vi "Main.vi"() -> ()   [LabVIEW 2015]
doc: "This example performs writes and reads on a serial port, as directed by the user. You can press the Write and Read buttons, and change the Read Count, while the example is running.\n\nThe parameters set for the serial port must match the parameters of the connected instrument or device. In this example, the Read Count parameter specifies the number of bytes that the serial port reads. If there were more bytes at the port than the specified number, those bytes would not be read. If there were less bytes at the port than the specified number, you would receive a timeout error.\n\nThis example expands upon the flow control options for XON and XOFF, allowing the user to choose those control characters. Also, the user can enable or disable a termination character. Some devices require a termination character in order to identify the end of command strings. Some devices send a termination character to signify the end of data to be read. This example shows how you can end the Read operation once a termination character is detected in the buffer and/or append a termination character at the end of the Write data."
uses:
  MPU-6050_states_machine_state.ctl
  <vilib>/Instr/_visa.llb/VISA Configure Serial Port (Instr).vi
panel:
  out "appended array":dbl[][](array[numeric])
  out "spreadsheet string":string
  out "x":dbl
  out "y":dbl
  out "z":dbl
  out "Pitch":dbl(knob) scale=0.0..360.0
  out "Roll":dbl(knob) scale=0.0..360.0
  out "Yaw":dbl(knob) scale=0.0..360.0
  out "read buffer":string
  in  "Save":bool
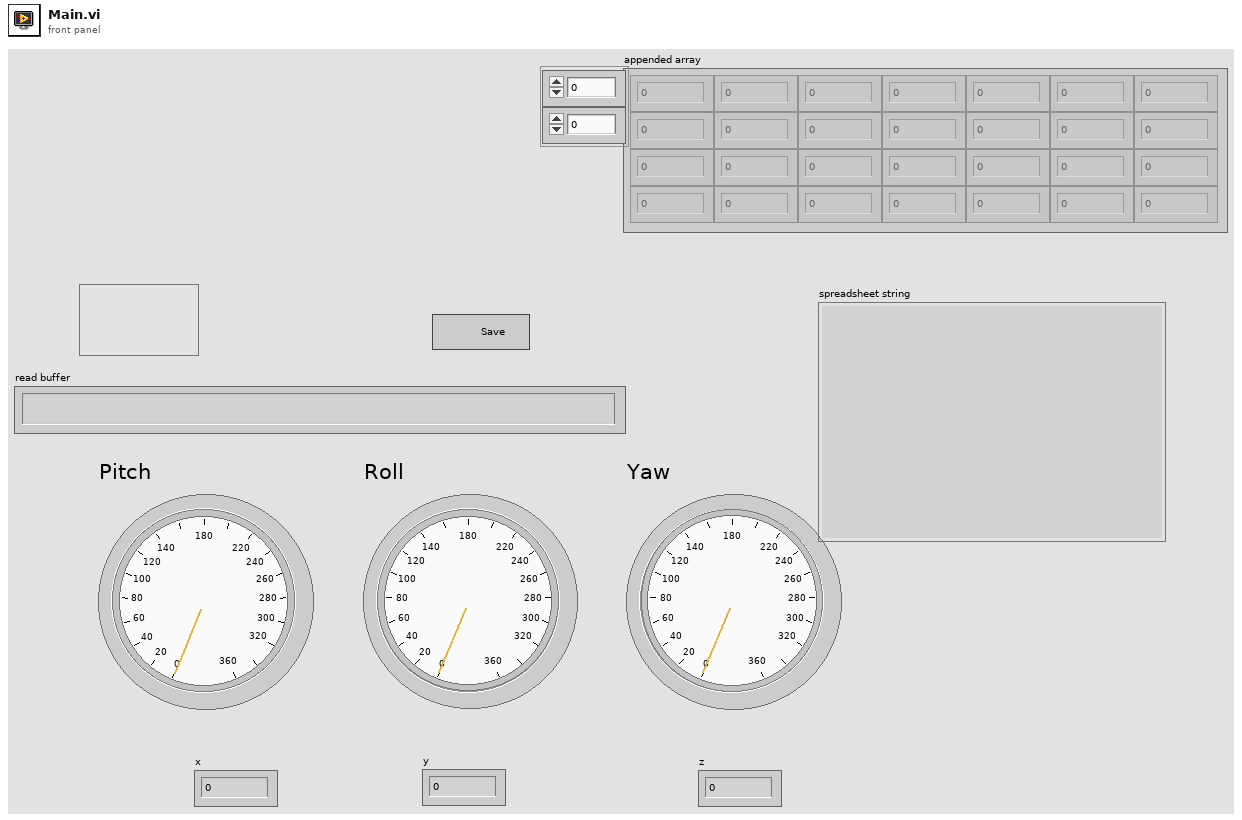
[diagram p1: front panel]
types:
  T1 = typedef "MPU-6050_states_machine_state.ctl" = enum16{"Initialize", "Calibrate", "Read", "Save", "Close", "Stop"}
  T2 = cluster{"VISA resource name":refnum<visa-resource-name>, "baud rate (9600)":u32, "Read buffer":string, "Byte count":u32, "GyroZ_bias":dbl, "GyraY_bias":dbl, "AccelX_bias":dbl, "AccelY_bias":dbl, "AccelZ_bias":dbl, "GyroX_bias":dbl, "Measurements":dbl[][]}
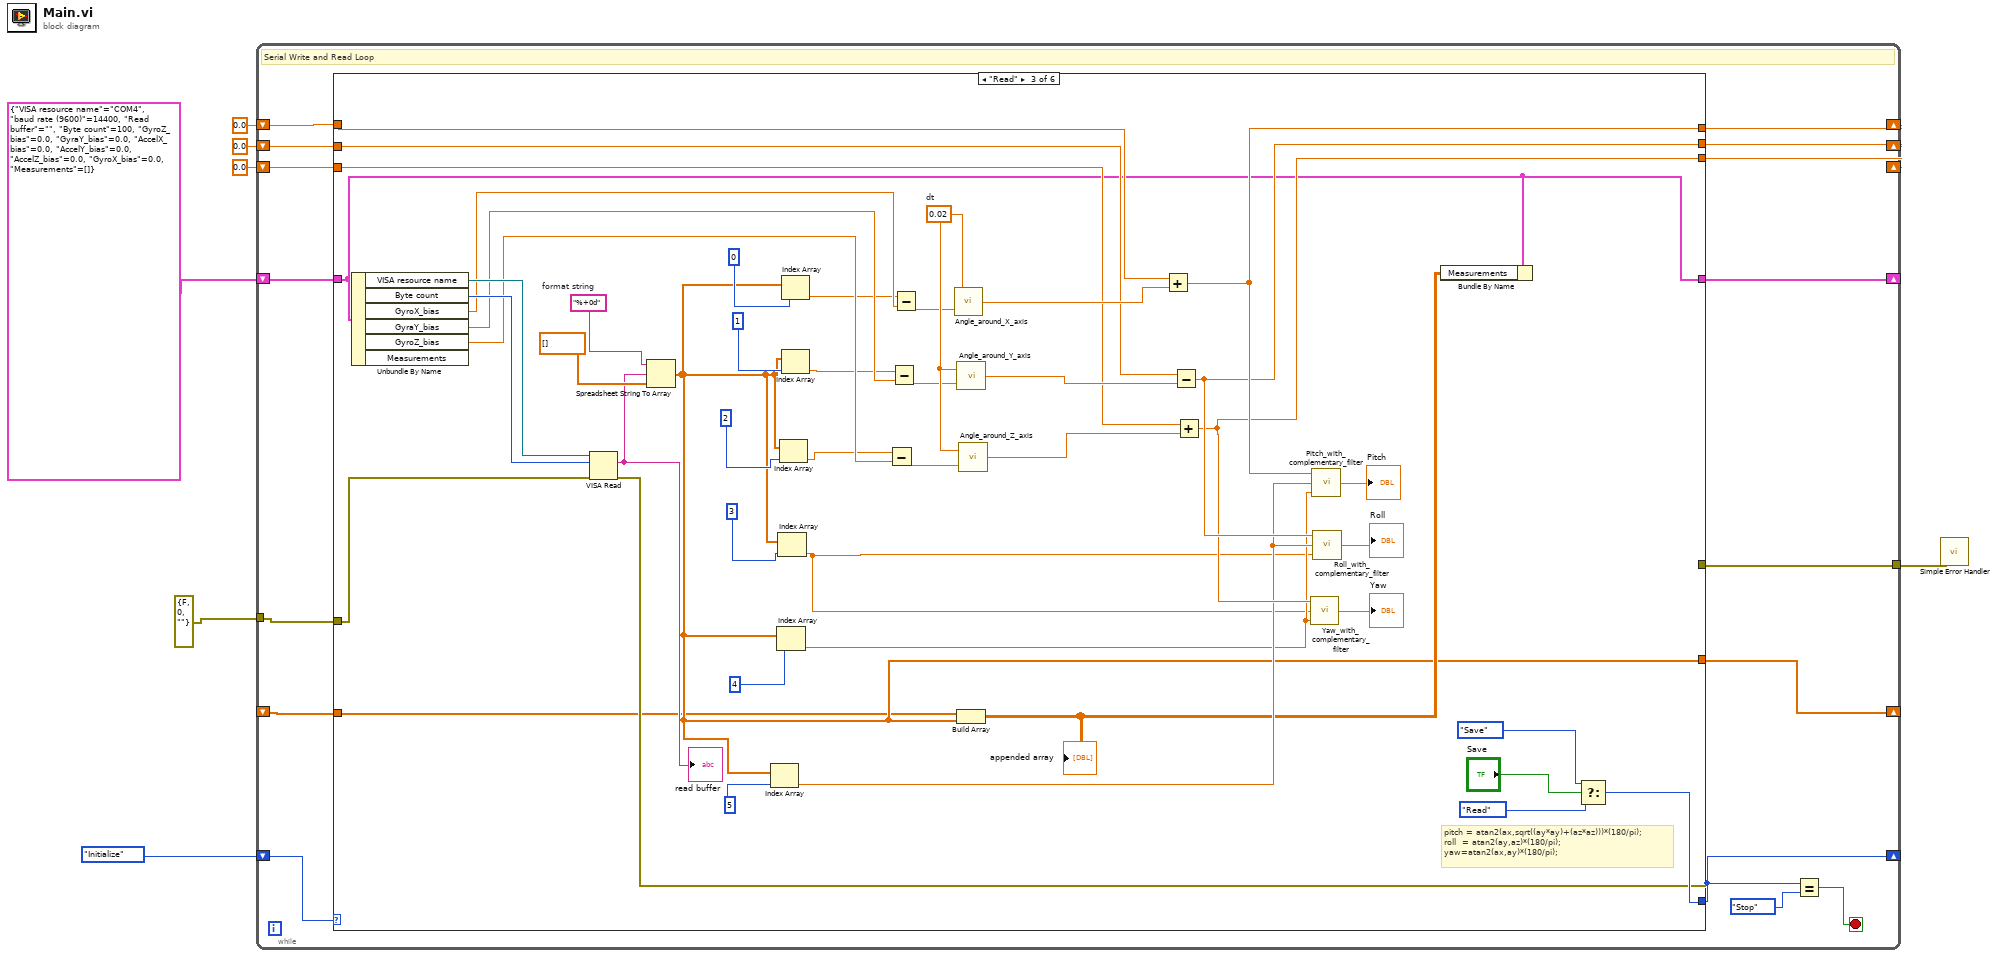
[diagram p0: block diagram]
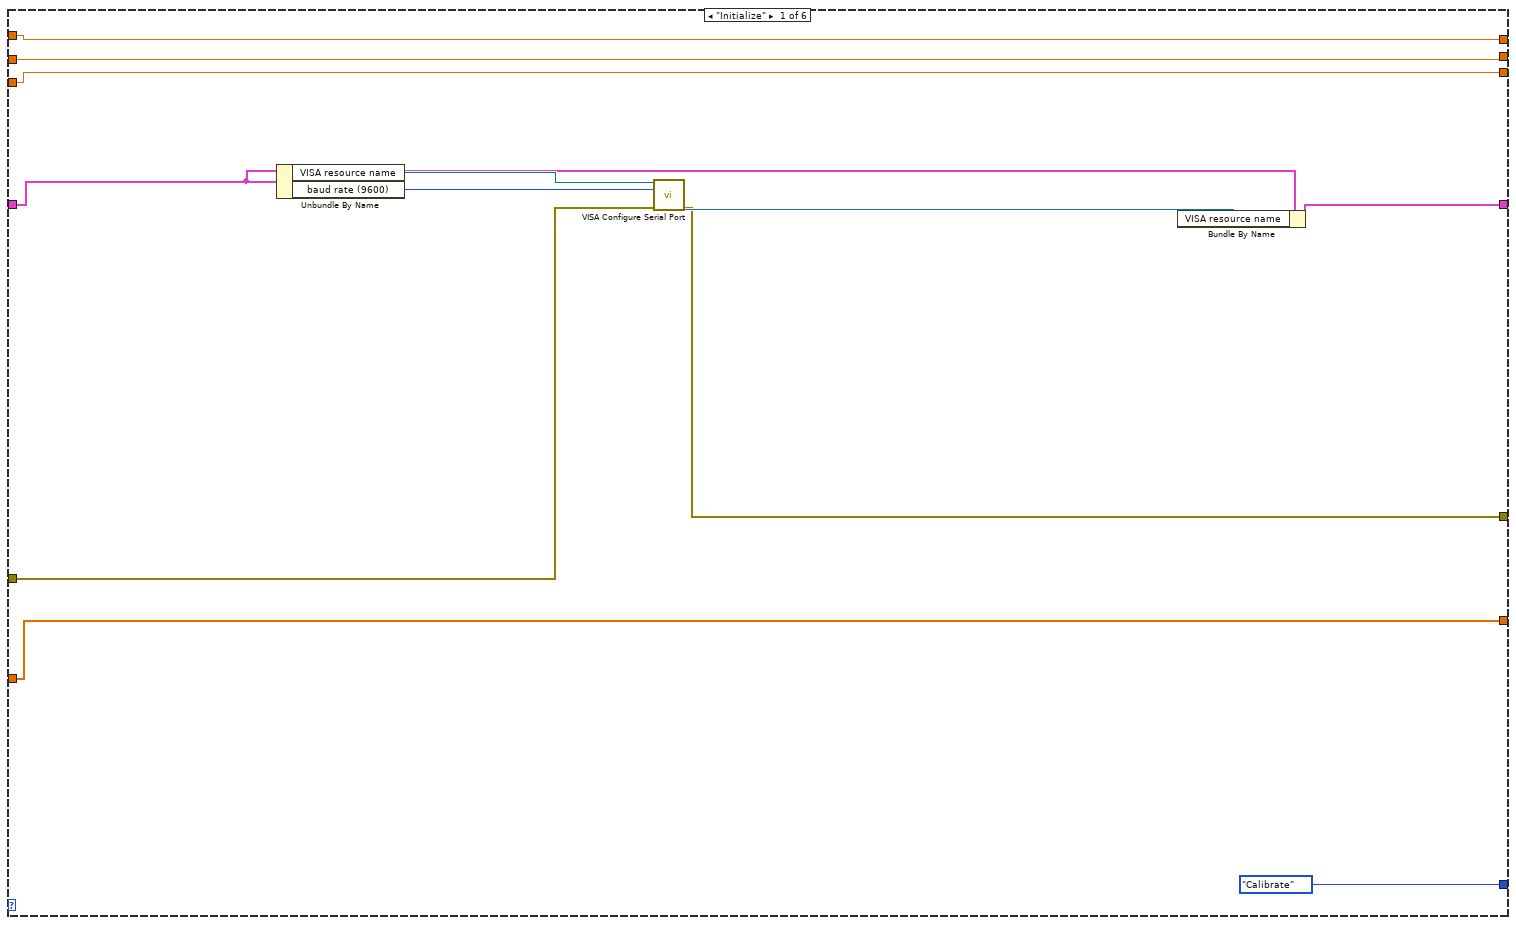
[diagram p2: hidden frame]
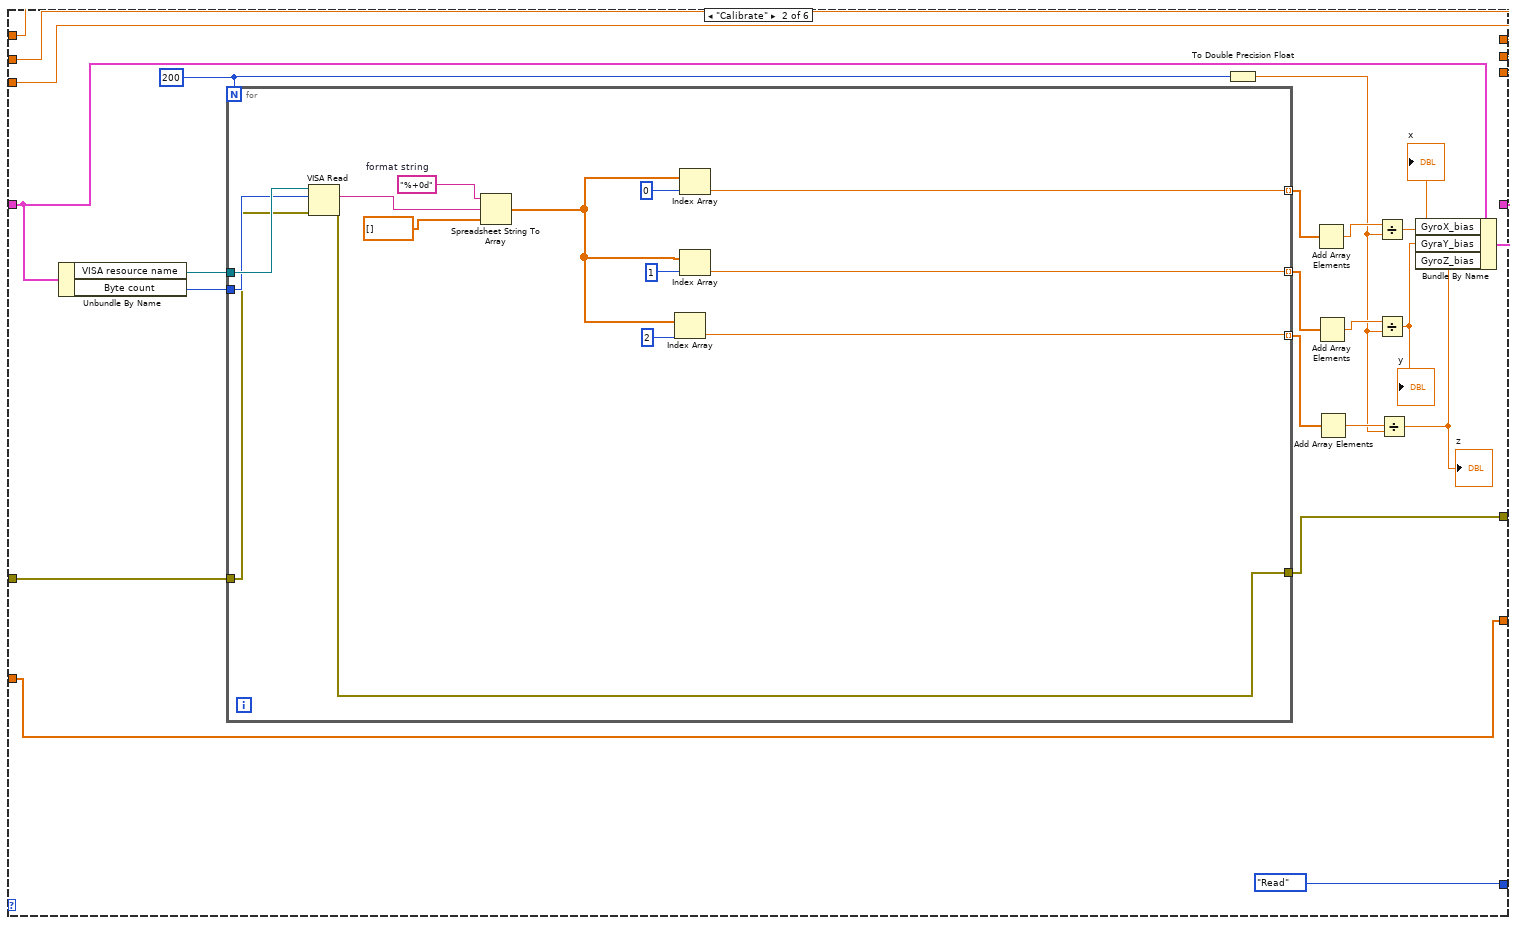
[diagram p3: hidden frame]
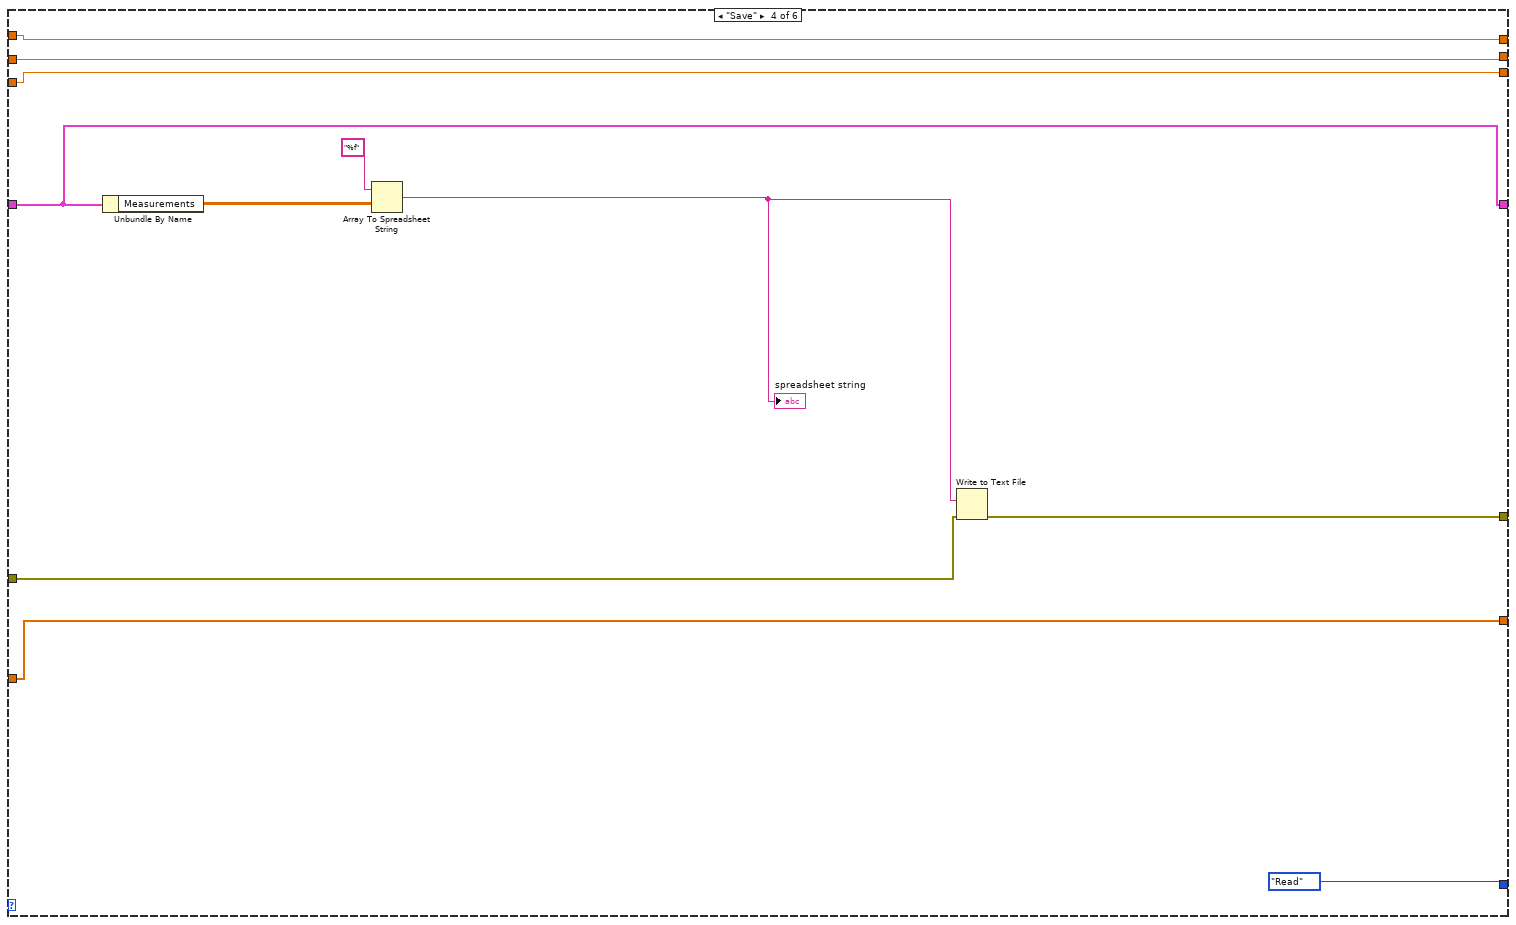
[diagram p4: hidden frame]
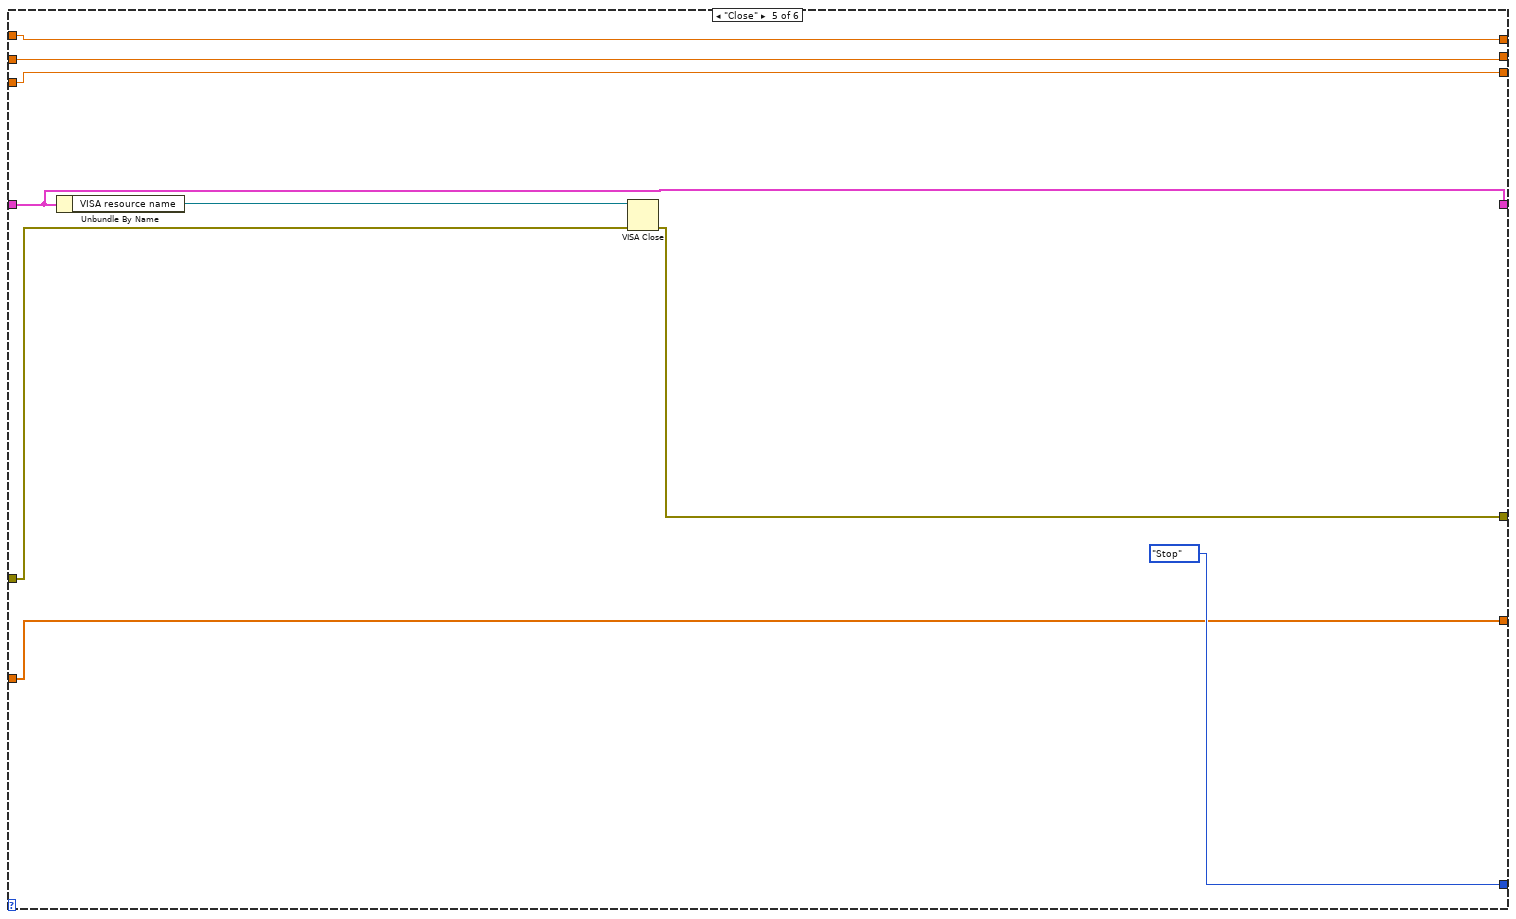
[diagram p5: hidden frame]
diagram:
  n1 = while {
    shift-right: [w15] -> _
    shift-left: T2 {"VISA resource name"="COM4", "baud rate (9600)"=14400, "Read buffer"="", "Byte count"=100, "GyroZ_bias"=0.0, "GyraY_bias"=0.0, "AccelX_bias"=0.0, "AccelY_bias"=0.0, "AccelZ_bias"=0.0, "GyroX_bias"=0.0, "Measurements"=[]} -> [w23]
    shift-right: [w22] -> _
    shift-left: 0.0 -> [w21]
    shift-right: [w20] -> _
    shift-left: 0.0 -> [w19]
    shift-right: [w18] -> _
    shift-left: 0.0 -> [w17]
    tunnel: errorcluster {"status"=FALSE, "code"=0, "source"=""} ("error in (no error)") -> [w16]
    shift-right: [w12] -> _
    shift-left: MPU-6050_states_machine_state."Initialize" -> [w14]
    tunnel: [w13] -> w4
    shift-right: [w9] -> _
    shift-left: _ -> [w8]
    stop <- w10 stop-if-true
    # "Serial Write and Read Loop"
    n2 = case shown="\"Read\"" w14 {
      selector: w14 -> [_ _ _ _ _ w139]
      tunnel: w23 -> [w32 w44 w76 w123 w132 w141]
      tunnel: [w28 w56 w107 w124 w137 w144] -> w22
      tunnel: w21 -> [w28 w56 w108 w124 w137 w144]
      tunnel: [w27 w55 w104 w125 w136 w143] -> w20
      tunnel: w19 -> [w27 w55 w105 w125 w136 w143]
      tunnel: [w26 w54 w101 w126 w135 w142] -> w18
      tunnel: w17 -> [w26 w54 w102 w126 w135 w142]
      tunnel: w16 -> [w35 w51 w93 w128 w133 w140]
      tunnel: [w30 w43 w76 w123 w132 w141] -> w15
      tunnel: [MPU-6050_states_machine_state."Calibrate" MPU-6050_states_machine_state."Read" w94 MPU-6050_states_machine_state."Read" MPU-6050_states_machine_state."Stop" w139] -> w12
      tunnel: [w25 w50 w92 w127 w131 w140] -> w13
      tunnel: [w24 w36 w73 w118 w129 w138] -> w9
      tunnel: w8 -> [w24 w36 w72 w118 w129 w138]
      frame "Initialize" {
        n3 = Unbundle By Name(w32) -> ("VISA resource name"=w34:refnum<visa-resource-name>, "baud rate (9600)"=w33:u32)
        n4 = call-poly "VISA Configure Serial Port"("VISA resource name"=w34, "baud rate (9600)"=w33, "error in (no error)"=w35) -> ("VISA resource name out"=w31:refnum<visa-resource-name>, "error out"=w25:errorcluster)  [unwired: 11 in]
        n5 = Bundle By Name(cluster=w32, "VISA resource name"=w31) -> (w30:T2)
      }
      frame "Calibrate" {
        w49 = 200
        n6 = Unbundle By Name(w44) -> ("VISA resource name"=w53:refnum<visa-resource-name>, "Byte count"=w52:u32)
        n7 = for {
          N: w49 -> [_]
          tunnel: w53 -> [w71]
          tunnel: w52 -> [w70]
          tunnel: w51 -> [w69]
          tunnel: [w68] -> w50
          tunnel: [w60] -> w39 mode=indexing
          tunnel: [w59] -> w38 mode=indexing
          tunnel: [w58] -> w37 mode=indexing
          w66 = "%+0d"  # format string
          n8 = VISA Read(VISA resource name=w71, byte count=w70, error in (no error)=w69) -> (read buffer=w65:string, error out=w68:errorcluster)  [unwired: 2 out]
          n9 = Spreadsheet String To Array(format string=w66, spreadsheet string=w65, array type (2D Dbl)=dbl[] []) -> (array=w61:dbl[])  [unwired: 1 in]
          n10 = Index Array "Index Array"(array=w61, index=2) -> (element=w58:dbl)
          n11 = Index Array "Index Array"(array=w61, index=0) -> (element=w60:dbl)
          n12 = Index Array "Index Array"(array=w61, index=1) -> (element=w59:dbl)
        }
        n13 = To Double Precision Float(number=w49) -> (double precision float=w45:dbl)
        n14 = Add Array Elements(numeric array=w39) -> (sum=w47:dbl)
        n15 = Add Array Elements(numeric array=w38) -> (sum=w48:dbl)
        n16 = Add Array Elements(numeric array=w37) -> (sum=w46:dbl)
        n17 = Divide(x=w47, y=w45) -> (x/y=w42:dbl)
        "x" <- w42
        n18 = Divide(x=w48, y=w45) -> (x/y=w41:dbl)
        "y" <- w41
        n19 = Divide(x=w46, y=w45) -> (x/y=w40:dbl)
        "z" <- w40
        n20 = Bundle By Name(cluster=w44, "GyroX_bias"=w42, "GyraY_bias"=w41, "GyroZ_bias"=w40) -> (w43:T2)
      }
      frame "Read" {
        w100 = 0.02  # dt
        w117 = "%+0d"  # format string
        # "pitch = atan2(ax,sqrt((ay*ay)+(az*az)))*(180/pi);\nroll  = atan2(ay,az)*(180/pi);\nyaw=atan2(ax,ay)*(180/pi);"
        n21 = Unbundle By Name(w76) -> ("VISA resource name"=w99:refnum<visa-resource-name>, "Byte count"=w98:u32, "GyroX_bias"=w85:dbl, "GyraY_bias"=w84:dbl, "GyroZ_bias"=w83:dbl)  [unwired: 1 out]
        n22 = VISA Read(VISA resource name=w99, byte count=w98, error in (no error)=w93) -> (read buffer=w75:string, error out=w92:errorcluster)  [unwired: 2 out]
        "read buffer" <- w75
        n23 = Spreadsheet String To Array(format string=w117, spreadsheet string=w75, array type (2D Dbl)=dbl[] []) -> (array=w73:dbl[])  [unwired: 1 in]
        n24 = Index Array "Index Array"(array=w73, index=5) -> (element=w80:dbl)
        n25 = Index Array "Index Array"(array=w73, index=4) -> (element=w78:dbl)
        n26 = Index Array "Index Array"(array=w73, index=3) -> (element=w77:dbl)
        n27 = Index Array "Index Array"(array=w73, index=2) -> (element=w81:dbl)
        n28 = Index Array "Index Array"(array=w73, index=0) -> (element=w82:dbl)
        n29 = Index Array "Index Array"(array=w73, index=1) -> (element=w79:dbl)
        n30 = Subtract(x=w81, y=w83) -> (x-y=w86:dbl)
        n31 = Subtract(x=w79, y=w84) -> (x-y=w87:dbl)
        n32 = Subtract(x=w82, y=w85) -> (x-y=w88:dbl)
        n33 = call "Angle_around_X_axis.vi"("gx"=w88, "dt"=w100) -> ("Angle around the X-axis (*pitch)"=w109:dbl)
        n34 = call "Angle_around_Y_axis.vi"("gy"=w87, "dt"=w100) -> ("Angle around the Y-axis (*roll)"=w106:dbl)
        n35 = Build Array(w72, w73) -> (w74:dbl[][])
        "appended array" <- w74
        n36 = call "Angle_around_Z_axis.vi"("gz"=w86, "dt"=w100) -> ("Angle around the Z-axis (*yaw)"=w103:dbl)
        n37 = Add(x=w108, y=w109) -> (x+y=w107:dbl)
        n38 = Subtract(x=w105, y=w106) -> (x-y=w104:dbl)
        n39 = Add(x=w102, y=w103) -> (x+y=w101:dbl)
        n40 = call "Yaw_with_complementary_filter.vi"("ay"=w78, "ax"=w77, "*yaw"=w101) -> ("yaw"=→"Yaw":dbl)
        n41 = call "Pitch_with_complementary_filter.vi"("ay"=w78, "az"=w80, "*pitch"=w107) -> ("pitch"=→"Pitch":dbl)
        n42 = call "Roll_with_complementary_filter.vi"("ax"=w77, "az"=w80, "*roll"=w104) -> ("roll"=→"Roll":dbl)
        n43 = Bundle By Name(cluster=w76, "Measurements"=w74) -> ()  [unwired: 1 out]
        n44 = Select(t=MPU-6050_states_machine_state."Save", s="Save", f=MPU-6050_states_machine_state."Read") -> (s? t:f=w94:T1)
      }
      frame "Save" {
        n45 = Unbundle By Name(w123) -> ("Measurements"=w121:dbl[][])
        n46 = Array To Spreadsheet String(array=w121, 3:"%f" ("format string")) -> (spreadsheet string=w119:string)  [unwired: 1 in]
        "spreadsheet string" <- w119
        n47 = Write to Text File(text=w119, error in=w128) -> (error out=w127:errorcluster)  [unwired: 2 in, 2 out]
      }
      frame "Close" {
        n48 = Unbundle By Name(w132) -> ("VISA resource name"=w134:refnum<visa-resource-name>)
        n49 = VISA Close(VISA resource name=w134, error in (no error)=w133) -> (error out=w131:errorcluster)
      }
      frame "Stop" {
      }
    }
    n50 = Equal?(x=w12, y=MPU-6050_states_machine_state."Stop") -> (x = y?=w10:bool)
  }
  n51 = call <vilib>:"Simple Error Handler.vi"("error in (no error)"=w4) -> ()  [unwired: 1 in, 8 out]
